vi "Write DELTA.vi"(8 "error in (no error)":errorcluster, 10 "Real Matrix":T1, 11 "Kalman Filter in":refnum<class "Kalman Filter.lvclass">) -> (0 "error out":errorcluster, 3 "Kalman Filter out":refnum<class "Kalman Filter.lvclass">)   [LabVIEW 2014, in "Observer Library.lvlib" / "Kalman Filter.lvclass"]
uses:
  Kalman Filter.lvclass
  <vilib>/Analysis/Matrix/Datatypes/RealMatrix.ctl
  Kalman Filter.lvclass/Kalman Filter.ctl
  <vilib>/Analysis/Matrix/NI_Matrix.lvlib
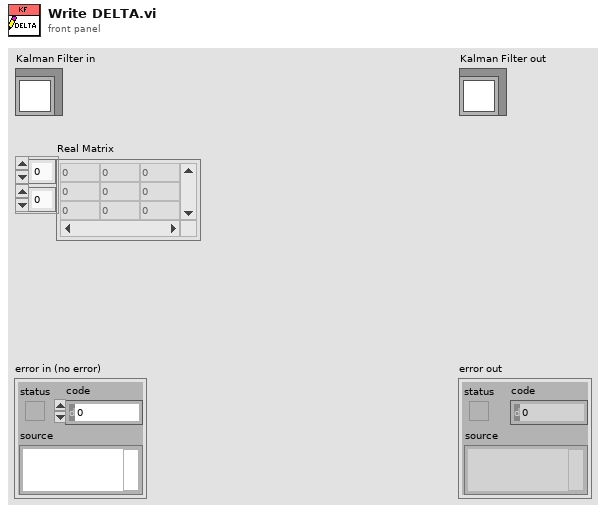
[diagram p1: front panel]
types:
  T1 = typedef "NI_Matrix.lvlib/RealMatrix.ctl" = dbl[][]
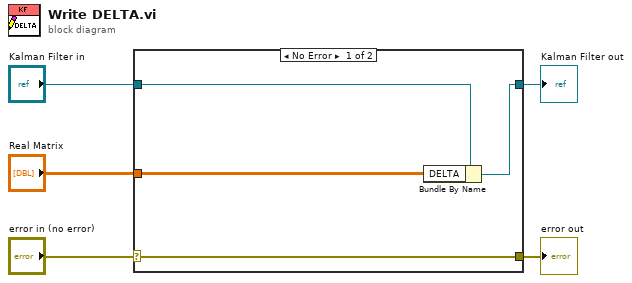
[diagram p0: block diagram]
diagram:
  n1 = case shown="No Error" "error in (no error)" {
    selector: "error in (no error)" -> [w9 w10]
    tunnel: [w9 w10] -> w4
    tunnel: [w7 w11] -> w2
    tunnel: "Kalman Filter in" -> [w8 w11]
    tunnel: "Real Matrix" -> [w6 _]
    frame No Error {
      n2 = Bundle By Name(cluster=w8, "DELTA"=w6) -> (w7:refnum<class "Kalman Filter.lvclass">)
    }
    frame Error {
    }
  }
  "error out" <- w4
  "Kalman Filter out" <- w2
